vi "SUB_Parsing_from_table_to_cluster.vi"(0 "ROM Table":string[][](table)=[["Device ID", "4294967295", "MAX Value: 4294967295 (FFFFFFFFh)"], ["YEAR", "255", "Year: 2255, MAX Value: 255 (FFh)"], ["Month", "255", "Month: 255, MAX Value: 255 (FFh)"], ["Day", "255", "Day: 255, MAX Value: 255 (FFh)"], ["Device Type", "65535", "-"], ["Manufacturer ID", "4294967295", "MAX Value: 4294967295 (FFFFFFFFh)"], ["Cal_Scale A", "0", "MAX Value: 255 (FF)"], ["Cal_Scale B", "0", "MAX Value: 255 (FF)"], ["Cal_Acc. X", "0", "-"], ["Cal_Acc. Y", "0", "-"], ["Cal_Acc. Z", "0", "-"], ["Cal_Gy. X", "0", "-"], ["Cal_Gy. Y", "0", "-"], ["Cal_Gy. Z", "0", "-"], ["Cal_Vol H", "0", "-"], ["Cal_Vol L", "0", "-"], ["Cal_CDC Off 1", "0", "-"], ["Cal_CDC Off 2", "0", "-"], ["Cal_CDC Off 3", "0", "-"], ["Cal_CDC Off 4", "0", "-"], ["Cal_CDC Off 5", "0", "-"], ["Cal_CDC Off 6", "0", "-"], ["Cal_CDC Off 7", "0", "-"], ["Cal_CDC Off 8", "0", "-"], ["Firmware Revision", "-", "-"], ["Operative Side", "-", "-"], ["Cal_Compart. A_10", "-", "-"], ["Cal_Compart. B_10", "-", "-"], ["Reserved", "-", "-"], ["Cal_Compart. A_11", "-", "-"], ["Cal_Compart. B_11", "-", "-"], ["Cal_Compart. A_12", "-", "-"], ["Cal_Compart. B_12", "-", "-"], ["Cal_Compart. A_13", "-", "-"], ["Cal_Compart. B_13", "-", "-"], ["Cal_Compart. A_14", "-", "-"], ["Cal_Compart. B_14", "-", "-"], ["Cal_Compart. A_16", "-", "-"], ["Cal_Compart. B_16", "-", "-"], ["Reserved", "-", "-"], ["Acc. X_0 value", "-", "-"], ["Acc. Y_0 value", "-", "-"], ["Acc. Z_0 value", "-", "-"], ["Acc. X_45 value", "-", "-"], ["Acc. Y_45 value", "-", "-"], ["Acc. Z_45 value", "-", "-"], ["Reserved", "-", "-"], ["Acc. X_90 value", "-", "-"], ["Acc. Y_90 value", "-", "-"], ["Acc. Z_90 value", "-", "-"], ["Acc. X_180 value", "-", "-"], ["Acc. Y_180 value", "-", "-"], ["Acc. Z_180 value", "-", "-"], ["Reserved", "-", "-"], ["", "", ""], ["", "", ""], ["", "", ""], ["", "", ""], ["", "", ""], ["", "", ""], ["", "", ""], ["", "", ""], ["", "", ""], ["", "", ""], ["", "", ""], ["", "", ""], ["", "", ""], ["", "", ""], ["", "", ""]]) -> (11 "Acclerometer value(90, 180)":T1 {"Check sum" format="%x"; "Reserved_2" format="%x"; "Reserved_1" format="%x"; "second counter_2" format="%x"; "Acc. Z_90 val_L" format="%x"; "second counter_1" format="%x"; "Acc. Z_180 val_L" format="%x"; "Acc. Z_180 val_H" format="%x"; "Acc. Y_180 val_L" format="%x"; "Acc. Y_180 val_H" format="%x"; "Acc. X_180 val_L" format="%x"; "Acc. X_180 val_H" format="%x"; "Acc. Z_90 val_H" format="%x"; "Acc. Y_90 val_L" format="%x"; "Acc. Y_90 val_H" format="%x"; "Acc. X_90 val_L" format="%x"; "Acc. X_90 val_H" format="%x"; "Packet ID" format="%x"}, 12 "data4":T3 {"Check sum" format="%x"; "Reserved_8" format="%x"; "Reserved_7" format="%x"; "Reserved_6" format="%x"; "Cal_Compart. B_16_2" format="%x"; "Reserved_5" format="%x"; "Reserved_4" format="%x"; "Reserved_3" format="%x"; "Reserved_2" format="%x"; "Reserved_1" format="%x"; "Cal_Compart. B_16_4" format="%x"; "Cal_Compart. B_16_3" format="%x"; "Cal_Compart. B_16_1" format="%x"; "Cal_Compart. A_16_4" format="%x"; "Cal_Compart. A_16_3" format="%x"; "Cal_Compart. A_16_2" format="%x"; "Cal_Compart. A_16_1" format="%x"; "Packet ID" format="%x"}, 13 "Acclerometer value(0, 45)":T2 {"Check sum" format="%x"; "Reserved_4" format="%x"; "Reserved_3" format="%x"; "Reserved_2" format="%x"; "Acc. Z_0 val_L" format="%x"; "Reserved_1" format="%x"; "Acc. Z_45 val_L" format="%x"; "Acc. Z_45 val_H" format="%x"; "Acc. Y_45 val_L" format="%x"; "Acc. Y_45 val_H" format="%x"; "Acc. X_45 val_L" format="%x"; "Acc. X_45 val_H" format="%x"; "Acc. Z_0 val_H" format="%x"; "Acc. Y_0 val_L" format="%x"; "Acc. Y_0 val_H" format="%x"; "Acc. X_0 val_L" format="%x"; "Acc. X_0 val_H" format="%x"; "Packet ID" format="%x"}, 14 "Device information":T7 {"Check sum 2" format="%x"; "Device Type L" format="%x"; "Device Type H" format="%x"; "Check sum" format="%x"; "Scale B" format="%x"; "Scale A" format="%x"; "Manufacturer Lot ID 4" format="%x"; "Manufacturer Lot ID 3" format="%x"; "Manufacturer Lot ID 2" format="%x"; "Manufacturer Lot ID 1" format="%x"; "Day" format="%x"; "Month" format="%x"; "Year" format="%x"; "Device ID 4" format="%x"; "Device ID 3" format="%x"; "Device ID 2" format="%x"; "Device ID 1" format="%x"; "Packet ID" format="%x"}, 15 "Cal information":T9 {"Check sum" format="%x"; "Voltage L 2.8V" format="%x"; "Voltage H 2.8V" format="%x"; "Voltage L 3.1V" format="%x"; "Acc Z_L_Cal" format="%x"; "Voltage H 3.1V" format="%x"; "Gyro Z_L_Cal" format="%x"; "Gyro Z_H_Cal" format="%x"; "Gyro Y_L_Cal" format="%x"; "Gyro Y_H_Cal" format="%x"; "Gyro X_L_Cal" format="%x"; "Gyro X_H_Cal" format="%x"; "Acc Z_H_Cal" format="%x"; "Acc Y_L_Cal" format="%x"; "Acc Y_H_Cal" format="%x"; "Acc X_L_Cal" format="%x"; "Acc X_H_Cal" format="%x"; "Packet ID" format="%x"}, 16 "PCAP zero information":T8 {"Check sum" format="%x"; "Sensor 8_L" format="%x"; "Sensor 8_H" format="%x"; "Sensor 7_L" format="%x"; "Sensor 7_H" format="%x"; "Sensor 6_L" format="%x"; "Sensor 6_H" format="%x"; "Sensor 5_L" format="%x"; "Sensor 5_H" format="%x"; "Sensor 4_L" format="%x"; "Sensor 4_H" format="%x"; "Sensor 3_L" format="%x"; "Sensor 3_H" format="%x"; "Sensor 2_L" format="%x"; "Sensor 2_H" format="%x"; "Sensor 1_L" format="%x"; "Sensor 1_H" format="%x"; "Packet ID" format="%x"}, 17 "data1":T6 {"Check sum" format="%x"; "Reserved_6" format="%x"; "Reserved_5" format="%x"; "Reserved_4" format="%x"; "Cal_Compart. A_10_4" format="%x"; "Reserved_3" format="%x"; "Reserved_2" format="%x"; "Reserved_1" format="%x"; "Cal_Compart. B_10_4" format="%x"; "Cal_Compart. B_10_3" format="%x"; "Cal_Compart. B_10_2" format="%x"; "Cal_Compart. B_10_1" format="%x"; "Cal_Compart. A_10_3" format="%x"; "Cal_Compart. A_10_2" format="%x"; "Cal_Compart. A_10_1" format="%x"; "Operative Side" format="%x"; "Firmware Revision" format="%x"; "Packet ID" format="%x"}, 18 "data2":T5 {"Check sum" format="%x"; "Cal_Compart. B_12_4" format="%x"; "Cal_Compart. B_12_3" format="%x"; "Cal_Compart. B_12_2" format="%x"; "Cal_Compart. B_11_2" format="%x"; "Cal_Compart. B_12_1" format="%x"; "Cal_Compart. A_12_4" format="%x"; "Cal_Compart. A_12_3" format="%x"; "Cal_Compart. A_12_2" format="%x"; "Cal_Compart. A_12_1" format="%x"; "Cal_Compart. B_11_4" format="%x"; "Cal_Compart. B_11_3" format="%x"; "Cal_Compart. B_11_1" format="%x"; "Cal_Compart. A_11_4" format="%x"; "Cal_Compart. A_11_3" format="%x"; "Cal_Compart. A_11_2" format="%x"; "Cal_Compart. A_11_1" format="%x"; "Packet ID" format="%x"}, 19 "data3":T4 {"Check sum" format="%x"; "Cal_Compart. B_14_4" format="%x"; "Cal_Compart. B_14_3" format="%x"; "Cal_Compart. B_14_2" format="%x"; "Cal_Compart. B_13_2" format="%x"; "Cal_Compart. B_14_1" format="%x"; "Cal_Compart. A_14_4" format="%x"; "Cal_Compart. A_14_3" format="%x"; "Cal_Compart. A_14_2" format="%x"; "Cal_Compart. A_14_1" format="%x"; "Cal_Compart. B_13_4" format="%x"; "Cal_Compart. B_13_3" format="%x"; "Cal_Compart. B_13_1" format="%x"; "Cal_Compart. A_13_4" format="%x"; "Cal_Compart. A_13_3" format="%x"; "Cal_Compart. A_13_2" format="%x"; "Cal_Compart. A_13_1" format="%x"; "Packet ID" format="%x"})   [LabVIEW 2015]
uses:
  Cluster Type/Cal information.ctl
  Cluster Type/PCAP zero information.ctl
  Cluster Type/Device information.ctl
  Cluster Type/add data1.ctl
  Cluster Type/add data2.ctl
  Cluster Type/add data3.ctl
  Cluster Type/add data4.ctl
  Cluster Type/Acclerometer value(0, 45).ctl
  Cluster Type/Acclerometer value(90, 180).ctl
panel:
  out "32비트 정수":u8
  out "32비트 정수 2":u8
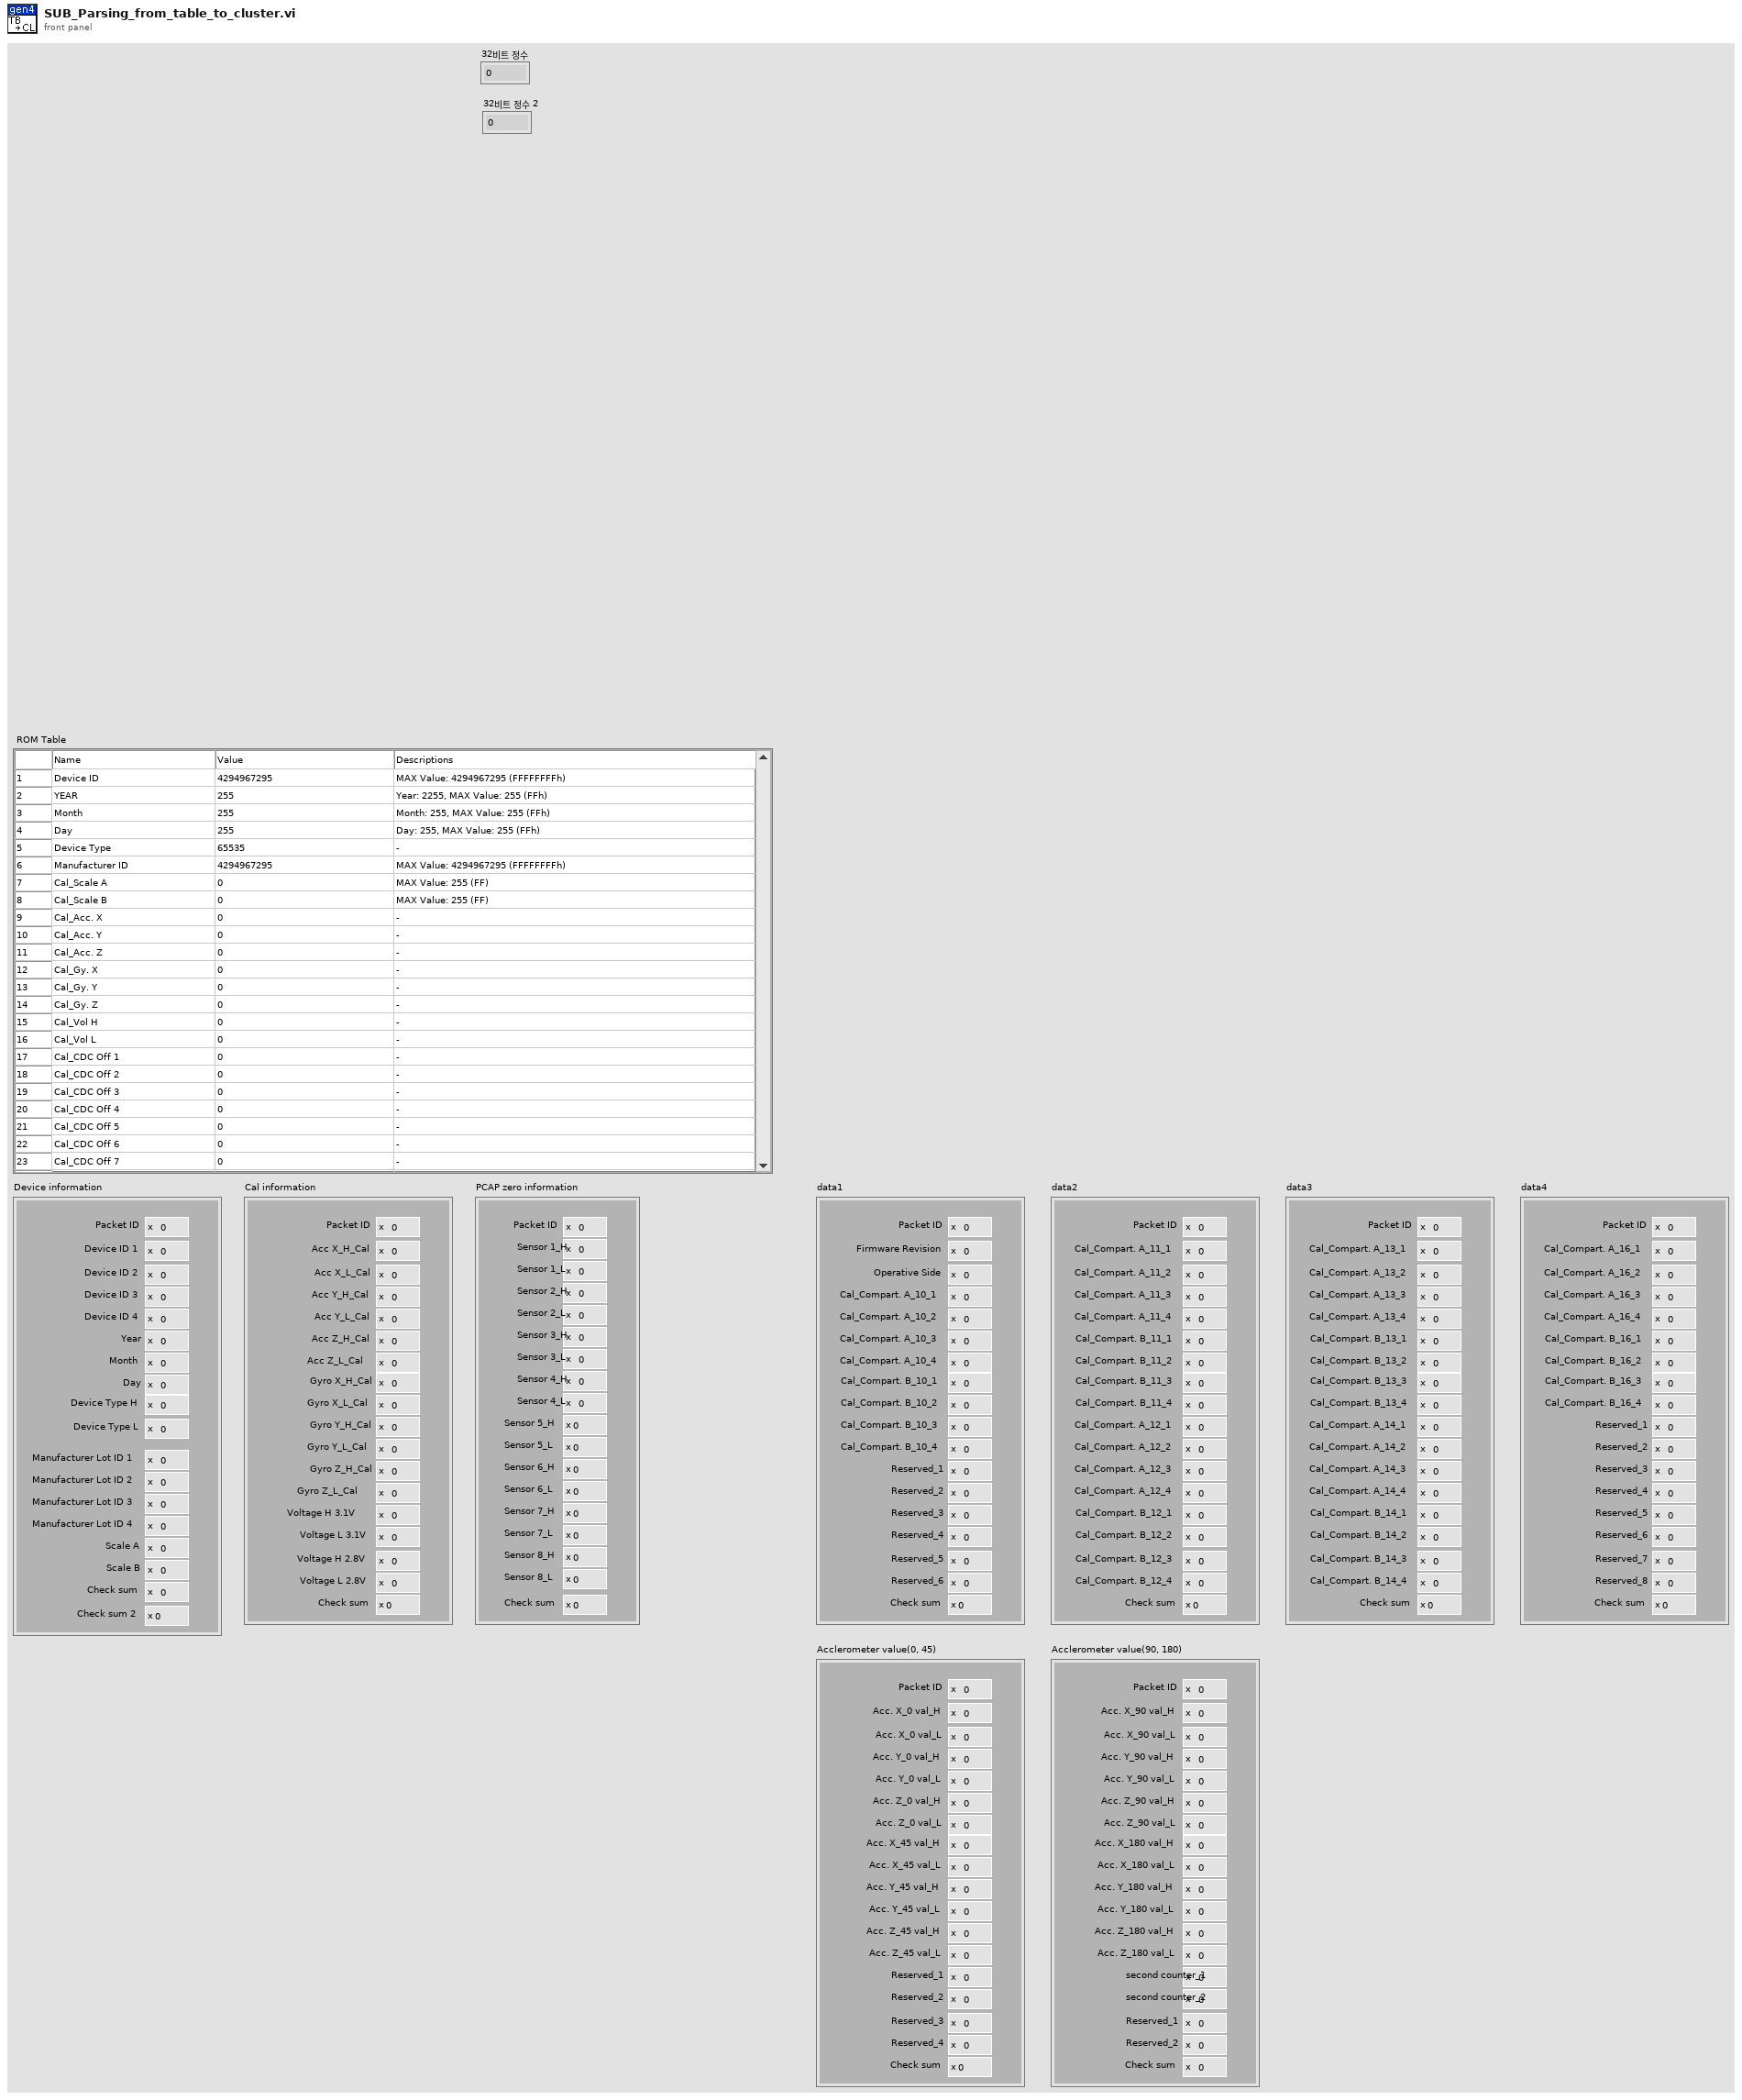
[diagram p1: front panel]
types:
  T1 = typedef "Acclerometer value(90, 180).ctl" = cluster{"Packet ID":u8, "Acc. X_90 val_H":u8, "Acc. X_90 val_L":u8, "Acc. Y_90 val_H":u8, "Acc. Y_90 val_L":u8, "Acc. Z_90 val_H":u8, "Acc. Z_90 val_L":u8, "Acc. X_180 val_H":u8, "Acc. X_180 val_L":u8, "Acc. Y_180 val_H":u8, "Acc. Y_180 val_L":u8, "Acc. Z_180 val_H":u8, "Acc. Z_180 val_L":u8, "second counter_1":u8, "second counter_2":u8, "Reserved_1":u8, "Reserved_2":u8, "Check sum":u8}
  T2 = typedef "Acclerometer value(0, 45).ctl" = cluster{"Packet ID":u8, "Acc. X_0 val_H":u8, "Acc. X_0 val_L":u8, "Acc. Y_0 val_H":u8, "Acc. Y_0 val_L":u8, "Acc. Z_0 val_H":u8, "Acc. Z_0 val_L":u8, "Acc. X_45 val_H":u8, "Acc. X_45 val_L":u8, "Acc. Y_45 val_H":u8, "Acc. Y_45 val_L":u8, "Acc. Z_45 val_H":u8, "Acc. Z_45 val_L":u8, "Reserved_1":u8, "Reserved_2":u8, "Reserved_3":u8, "Reserved_4":u8, "Check sum":u8}
  T3 = typedef "add data4.ctl" = cluster{"Packet ID":u8, "Cal_Compart. A_16_1":u8, "Cal_Compart. A_16_2":u8, "Cal_Compart. A_16_3":u8, "Cal_Compart. A_16_4":u8, "Cal_Compart. B_16_1":u8, "Cal_Compart. B_16_2":u8, "Cal_Compart. B_16_3":u8, "Cal_Compart. B_16_4":u8, "Reserved_1":u8, "Reserved_2":u8, "Reserved_3":u8, "Reserved_4":u8, "Reserved_5":u8, "Reserved_6":u8, "Reserved_7":u8, "Reserved_8":u8, "Check sum":u8}
  T4 = typedef "add data3.ctl" = cluster{"Packet ID":u8, "Cal_Compart. A_13_1":u8, "Cal_Compart. A_13_2":u8, "Cal_Compart. A_13_3":u8, "Cal_Compart. A_13_4":u8, "Cal_Compart. B_13_1":u8, "Cal_Compart. B_13_2":u8, "Cal_Compart. B_13_3":u8, "Cal_Compart. B_13_4":u8, "Cal_Compart. A_14_1":u8, "Cal_Compart. A_14_2":u8, "Cal_Compart. A_14_3":u8, "Cal_Compart. A_14_4":u8, "Cal_Compart. B_14_1":u8, "Cal_Compart. B_14_2":u8, "Cal_Compart. B_14_3":u8, "Cal_Compart. B_14_4":u8, "Check sum":u8}
  T5 = typedef "add data2.ctl" = cluster{"Packet ID":u8, "Cal_Compart. A_11_1":u8, "Cal_Compart. A_11_2":u8, "Cal_Compart. A_11_3":u8, "Cal_Compart. A_11_4":u8, "Cal_Compart. B_11_1":u8, "Cal_Compart. B_11_2":u8, "Cal_Compart. B_11_3":u8, "Cal_Compart. B_11_4":u8, "Cal_Compart. A_12_1":u8, "Cal_Compart. A_12_2":u8, "Cal_Compart. A_12_3":u8, "Cal_Compart. A_12_4":u8, "Cal_Compart. B_12_1":u8, "Cal_Compart. B_12_2":u8, "Cal_Compart. B_12_3":u8, "Cal_Compart. B_12_4":u8, "Check sum":u8}
  T6 = typedef "add data1.ctl" = cluster{"Packet ID":u8, "Firmware Revision":u8, "Operative Side":u8, "Cal_Compart. A_10_1":u8, "Cal_Compart. A_10_2":u8, "Cal_Compart. A_10_3":u8, "Cal_Compart. A_10_4":u8, "Cal_Compart. B_10_1":u8, "Cal_Compart. B_10_2":u8, "Cal_Compart. B_10_3":u8, "Cal_Compart. B_10_4":u8, "Reserved_1":u8, "Reserved_2":u8, "Reserved_3":u8, "Reserved_4":u8, "Reserved_5":u8, "Reserved_6":u8, "Check sum":u8}
  T7 = typedef "Device information.ctl" = cluster{"Packet ID":u8, "Device ID 1":u8, "Device ID 2":u8, "Device ID 3":u8, "Device ID 4":u8, "Year":u8, "Month":u8, "Day":u8, "Device Type H":u8, "Device Type L":u8, "Manufacturer Lot ID 1":u8, "Manufacturer Lot ID 2":u8, "Manufacturer Lot ID 3":u8, "Manufacturer Lot ID 4":u8, "Scale A":u8, "Scale B":u8, "Check sum":u8, "Check sum 2":u8}
  T8 = typedef "PCAP zero information.ctl" = cluster{"Packet ID":u8, "Sensor 1_H":u8, "Sensor 1_L":u8, "Sensor 2_H":u8, "Sensor 2_L ":u8, "Sensor 3_H":u8, "Sensor 3_L":u8, "Sensor 4_H":u8, "Sensor 4_L":u8, "Sensor 5_H":u8, "Sensor 5_L":u8, "Sensor 6_H":u8, "Sensor 6_L":u8, "Sensor 7_H":u8, "Sensor 7_L":u8, "Sensor 8_H":u8, "Sensor 8_L":u8, "Check sum":u8}
  T9 = typedef "Cal information.ctl" = cluster{"Packet ID":u8, "Acc X_H_Cal":u8, "Acc X_L_Cal":u8, "Acc Y_H_Cal":u8, "Acc Y_L_Cal":u8, "Acc Z_H_Cal":u8, "Acc Z_L_Cal":u8, "Gyro X_H_Cal":u8, "Gyro X_L_Cal":u8, "Gyro Y_H_Cal":u8, "Gyro Y_L_Cal":u8, "Gyro Z_H_Cal":u8, "Gyro Z_L_Cal":u8, "Voltage H 3.1V":u8, "Voltage L 3.1V":u8, "Voltage H 2.8V":u8, "Voltage L 2.8V":u8, "Check sum":u8}
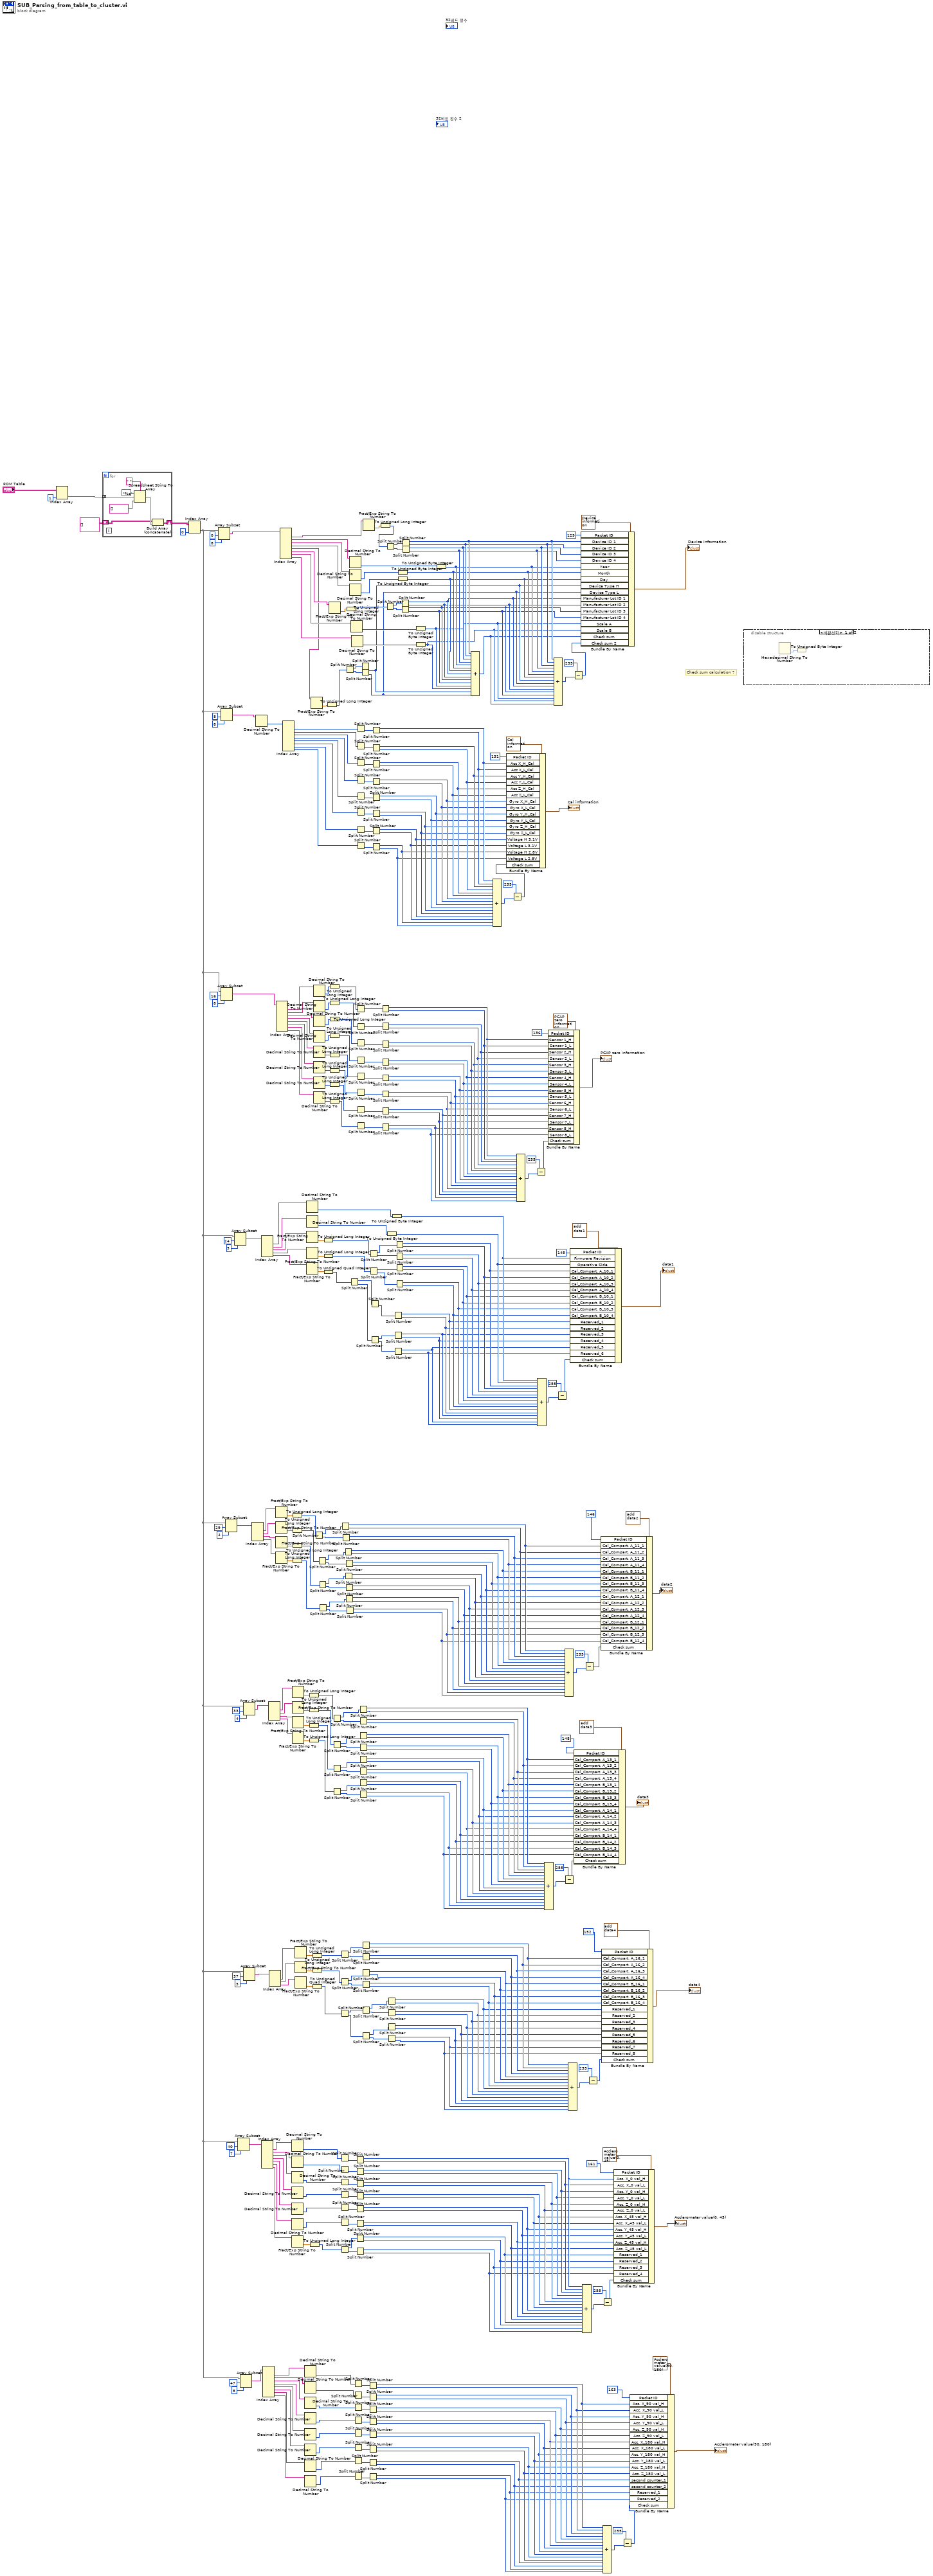
[diagram p0: block diagram]
diagram:
  # "Check sum calculation ?"
  n1 = Index Array(array="ROM Table", index (col)=1 ("비활성화된 인덱스 (열)")) -> (element=w388:string[])  [unwired: 1 in]
  n2 = for {
    tunnel: w388 -> [w441] mode=indexing
    shift-right: [w436] -> w385
    shift-left: string[][] [] -> [w435]
    n3 = Spreadsheet String To Array(delimiter (Tab)=" " ("구분 문자(탭)"), format string="%s" ("포맷 문자열"), spreadsheet string=w441, array type (2D Dbl)=string[] []) -> (array=w437:string[])
    n4 = Build Array (concatenate)(w435, w437) -> (w436:string[][])
  }
  n5 = Index Array(array=w385, index (col)=0 ("비활성화된 인덱스 (열)")) -> (element=w313:string[])  [unwired: 1 in]
  n6 = Array Subset(array=w313, index=0 ("인덱스"), length=8 ("길이")) -> (w417:string[])
  n7 = Array Subset(array=w313, index=8 ("인덱스"), length=8 ("길이")) -> (w412:string[])
  n8 = Array Subset(array=w313, index=16 ("인덱스"), length=8 ("길이")) -> (w236:string[])
  n9 = Array Subset(array=w313, index=29 ("인덱스"), length=4 ("길이")) -> (w196:string[])
  n10 = Array Subset(array=w313, index=24 ("인덱스"), length=5 ("길이")) -> (w227:string[])
  n11 = Array Subset(array=w313, index=40 ("인덱스"), length=7 ("길이")) -> (w81:string[])
  n12 = Array Subset(array=w313, index=47 ("인덱스"), length=8 ("길이")) -> (w28:string[])
  n13 = Array Subset(array=w313, index=33 ("인덱스"), length=4 ("길이")) -> (w156:string[])
  n14 = Array Subset(array=w313, index=37 ("인덱스"), length=3 ("길이")) -> (w130:string[])
  n15 = Index Array(array=w196) -> (element #1=w191:string, element #2=w190:string, element #3=w189:string, element #4=w188:string)  [unwired: 4 in]
  n16 = Decimal String To Number(string=w412) -> (number=w411:i32[])  [unwired: 2 in, 1 out]
  n17 = Index Array(array=w227) -> (element #1=w226:string, element #2=w225:string, element #3=w85:string, element #4=w84:string, element #5=w222:string)  [unwired: 5 in]
  n18 = Index Array(array=w81) -> (element #1=w80:string, element #2=w79:string, element #3=w78:string, element #4=w77:string, element #5=w76:string, element #6=w75:string, element #7=w73:string)  [unwired: 7 in]
  n19 = Index Array(array=w28) -> (element #1=w40:string, element #2=w39:string, element #3=w38:string, element #4=w37:string, element #5=w36:string, element #6=w35:string, element #7=w12:string, element #8=w11:string)  [unwired: 8 in]
  n20 = Index Array(array=w156) -> (element #1=w160:string, element #2=w159:string, element #3=w158:string, element #4=w157:string)  [unwired: 4 in]
  n21 = Index Array(array=w130) -> (element #1=w129:string, element #2=w128:string, element #3=w126:string)  [unwired: 3 in]
  n22 = Fract/Exp String To Number(string=w191) -> (number=w194:dbl)  [unwired: 3 in, 1 out]
  n23 = Fract/Exp String To Number(string=w190) -> (number=w195:dbl)  [unwired: 3 in, 1 out]
  n24 = Fract/Exp String To Number(string=w189) -> (number=w193:dbl)  [unwired: 3 in, 1 out]
  n25 = Fract/Exp String To Number(string=w188) -> (number=w192:dbl)  [unwired: 3 in, 1 out]
  n26 = Index Array(array=w236) -> (element #1=w235:string, element #2=w234:string, element #3=w233:string, element #4=w232:string, element #5=w231:string, element #6=w230:string, element #7=w229:string, element #8=w228:string)  [unwired: 8 in]
  n27 = Index Array(array=w417) -> (element #1=w378:string, element #2=w426:string, element #3=w425:string, element #4=w424:string, element #5=w372:string, element #6=w375:string, element #7=w383:string, element #8=w382:string)  [unwired: 8 in]
  n28 = Index Array(array=w411) -> (element #1=w410:i32, element #2=w404:i32, element #3=w403:i32, element #4=w400:i32, element #5=w399:i32, element #6=w398:i32, element #7=w397:i32, element #8=w396:i32)  [unwired: 8 in]
  n29 = To Unsigned Long Integer(number=w194) -> (unsigned 32bit integer=w187:u32)
  n30 = To Unsigned Long Integer(number=w195) -> (unsigned 32bit integer=w186:u32)
  n31 = To Unsigned Long Integer(number=w193) -> (unsigned 32bit integer=w185:u32)
  n32 = To Unsigned Long Integer(number=w192) -> (unsigned 32bit integer=w184:u32)
  n33 = Decimal String To Number(string=w80) -> (number=w72:i32)  [unwired: 2 in, 1 out]
  n34 = Decimal String To Number(string=w79) -> (number=w71:i32)  [unwired: 2 in, 1 out]
  n35 = Decimal String To Number(string=w78) -> (number=w70:i32)  [unwired: 2 in, 1 out]
  n36 = Decimal String To Number(string=w77) -> (number=w69:i32)  [unwired: 2 in, 1 out]
  n37 = Decimal String To Number(string=w76) -> (number=w68:i32)  [unwired: 2 in, 1 out]
  n38 = Decimal String To Number(string=w75) -> (number=w67:i32)  [unwired: 2 in, 1 out]
  n39 = Fract/Exp String To Number(string=w73) -> (number=w74:dbl)  [unwired: 3 in, 1 out]
  n40 = Fract/Exp String To Number(string=w160) -> (number=w163:dbl)  [unwired: 3 in, 1 out]
  n41 = Fract/Exp String To Number(string=w159) -> (number=w164:dbl)  [unwired: 3 in, 1 out]
  n42 = Fract/Exp String To Number(string=w158) -> (number=w162:dbl)  [unwired: 3 in, 1 out]
  n43 = Fract/Exp String To Number(string=w157) -> (number=w161:dbl)  [unwired: 3 in, 1 out]
  n44 = Fract/Exp String To Number(string=w129) -> (number=w131:dbl)  [unwired: 3 in, 1 out]
  n45 = Fract/Exp String To Number(string=w128) -> (number=w132:dbl)  [unwired: 3 in, 1 out]
  n46 = Fract/Exp String To Number(string=w126) -> (number=w127:dbl)  [unwired: 3 in, 1 out]
  n47 = Decimal String To Number(string=w40) -> (number=w34:i32)  [unwired: 2 in, 1 out]
  n48 = Decimal String To Number(string=w39) -> (number=w33:i32)  [unwired: 2 in, 1 out]
  n49 = Decimal String To Number(string=w38) -> (number=w32:i32)  [unwired: 2 in, 1 out]
  n50 = Decimal String To Number(string=w37) -> (number=w31:i32)  [unwired: 2 in, 1 out]
  n51 = Decimal String To Number(string=w36) -> (number=w30:i32)  [unwired: 2 in, 1 out]
  n52 = Decimal String To Number(string=w35) -> (number=w29:i32)  [unwired: 2 in, 1 out]
  n53 = Decimal String To Number(string=w12) -> (number=w10:i32)  [unwired: 2 in, 1 out]
  n54 = Decimal String To Number(string=w11) -> (number=w9:i32)  [unwired: 2 in, 1 out]
  n55 = Decimal String To Number(string=w226) -> (number=w224:i32)  [unwired: 2 in, 1 out]
  n56 = Decimal String To Number(string=w225) -> (number=w223:i32)  [unwired: 2 in, 1 out]
  n57 = Fract/Exp String To Number(string=w85) -> (number=w87:dbl)  [unwired: 3 in, 1 out]
  n58 = Fract/Exp String To Number(string=w84) -> (number=w86:dbl)  [unwired: 3 in, 1 out]
  n59 = Fract/Exp String To Number(string=w222) -> (number=w221:dbl)  [unwired: 3 in, 1 out]
  n60 = To Unsigned Long Integer(number=w163) -> (unsigned 32bit integer=w155:u32)
  n61 = To Unsigned Long Integer(number=w164) -> (unsigned 32bit integer=w154:u32)
  n62 = To Unsigned Long Integer(number=w162) -> (unsigned 32bit integer=w153:u32)
  n63 = To Unsigned Long Integer(number=w161) -> (unsigned 32bit integer=w152:u32)
  n64 = To Unsigned Long Integer(number=w74) -> (unsigned 32bit integer=w66:u32)
  n65 = Fract/Exp String To Number(string=w372) -> (number=w373:dbl)  [unwired: 3 in, 1 out]
  n66 = To Unsigned Long Integer(number=w131) -> (unsigned 32bit integer=w125:u32)
  n67 = To Unsigned Long Integer(number=w132) -> (unsigned 32bit integer=w124:u32)
  n68 = To Unsigned Quad Integer(1:w127) -> (0:w123:u64)
  n69 = Decimal String To Number(string=w235) -> (number=w103:i32)  [unwired: 2 in, 1 out]
  n70 = Decimal String To Number(string=w234) -> (number=w102:i32)  [unwired: 2 in, 1 out]
  n71 = Decimal String To Number(string=w233) -> (number=w101:i32)  [unwired: 2 in, 1 out]
  n72 = Decimal String To Number(string=w232) -> (number=w100:i32)  [unwired: 2 in, 1 out]
  n73 = Decimal String To Number(string=w231) -> (number=w99:i32)  [unwired: 2 in, 1 out]
  n74 = Decimal String To Number(string=w230) -> (number=w98:i32)  [unwired: 2 in, 1 out]
  n75 = Decimal String To Number(string=w229) -> (number=w97:i32)  [unwired: 2 in, 1 out]
  n76 = Decimal String To Number(string=w228) -> (number=w96:i32)  [unwired: 2 in, 1 out]
  n77 = Split Number(x=w187) -> (hi(x)=w358:u16, lo(x)=w359:u16)
  n78 = Split Number(x=w186) -> (hi(x)=w355:u16, lo(x)=w356:u16)
  n79 = Split Number(x=w185) -> (hi(x)=w353:u16, lo(x)=w354:u16)
  n80 = Split Number(x=w184) -> (hi(x)=w351:u16, lo(x)=w352:u16)
  n81 = To Unsigned Long Integer(number=w87) -> (unsigned 32bit integer=w83:u32)
  n82 = To Unsigned Long Integer(number=w86) -> (unsigned 32bit integer=w82:u32)
  n83 = To Unsigned Quad Integer(1:w221) -> (0:w220:u64)
  n84 = To Unsigned Long Integer(number=w373) -> (unsigned 32bit integer=w371:u32)
  n85 = Fract/Exp String To Number(string=w375) -> (number=w376:dbl)  [unwired: 3 in, 1 out]
  n86 = To Unsigned Long Integer(number=w103) -> (unsigned 32bit integer=w95:u32)
  n87 = To Unsigned Long Integer(number=w102) -> (unsigned 32bit integer=w94:u32)
  n88 = To Unsigned Long Integer(number=w101) -> (unsigned 32bit integer=w93:u32)
  n89 = To Unsigned Long Integer(number=w100) -> (unsigned 32bit integer=w92:u32)
  n90 = To Unsigned Long Integer(number=w99) -> (unsigned 32bit integer=w91:u32)
  n91 = To Unsigned Long Integer(number=w98) -> (unsigned 32bit integer=w90:u32)
  n92 = To Unsigned Long Integer(number=w97) -> (unsigned 32bit integer=w89:u32)
  n93 = To Unsigned Long Integer(number=w96) -> (unsigned 32bit integer=w88:u32)
  n94 = Split Number(x=w155) -> (hi(x)=w346:u16, lo(x)=w347:u16)
  n95 = Split Number(x=w154) -> (hi(x)=w344:u16, lo(x)=w345:u16)
  n96 = Split Number(x=w153) -> (hi(x)=w342:u16, lo(x)=w343:u16)
  n97 = Split Number(x=w152) -> (hi(x)=w340:u16, lo(x)=w341:u16)
  n98 = Split Number(x=w125) -> (hi(x)=w335:u16, lo(x)=w336:u16)
  n99 = Split Number(x=w124) -> (hi(x)=w333:u16, lo(x)=w334:u16)
  n100 = Split Number(x=w123) -> (hi(x)=w330:u32, lo(x)=w327:u32)
  n101 = Split Number(x=w72) -> (lo(x)=w323:u16)  [unwired: 1 out]
  n102 = Split Number(x=w71) -> (lo(x)=w322:u16)  [unwired: 1 out]
  n103 = Split Number(x=w70) -> (lo(x)=w321:u16)  [unwired: 1 out]
  n104 = Split Number(x=w69) -> (lo(x)=w320:u16)  [unwired: 1 out]
  n105 = Split Number(x=w68) -> (lo(x)=w319:u16)  [unwired: 1 out]
  n106 = Split Number(x=w67) -> (lo(x)=w318:u16)  [unwired: 1 out]
  n107 = Split Number(x=w66) -> (hi(x)=w316:u16, lo(x)=w317:u16)
  n108 = Split Number(x=w358) -> (hi(x)=w180:u8, lo(x)=w179:u8)
  n109 = Split Number(x=w359) -> (hi(x)=w178:u8, lo(x)=w177:u8)
  n110 = Split Number(x=w355) -> (hi(x)=w176:u8, lo(x)=w175:u8)
  n111 = Split Number(x=w353) -> (hi(x)=w172:u8, lo(x)=w171:u8)
  n112 = Split Number(x=w356) -> (hi(x)=w174:u8, lo(x)=w173:u8)
  n113 = Split Number(x=w351) -> (hi(x)=w168:u8, lo(x)=w167:u8)
  n114 = Split Number(x=w354) -> (hi(x)=w170:u8, lo(x)=w169:u8)
  n115 = Split Number(x=w371) -> (hi(x)=w421:u16, lo(x)=w420:u16)
  n116 = Split Number(x=w352) -> (hi(x)=w166:u8, lo(x)=w165:u8)
  n117 = To Unsigned Long Integer(number=w376) -> (unsigned 32bit integer=w374:u32)
  n118 = Split Number(x=w220) -> (hi(x)=w217:u32, lo(x)=w216:u32)
  n119 = Decimal String To Number(string=w426) -> (number=w384:i32)  [unwired: 2 in, 1 out]
  n120 = Decimal String To Number(string=w425) -> (number=w423:i32)  [unwired: 2 in, 1 out]
  n121 = Decimal String To Number(string=w424) -> (number=w422:i32)  [unwired: 2 in, 1 out]
  n122 = Decimal String To Number(string=w383) -> (number=w381:i32)  [unwired: 2 in, 1 out]
  n123 = Decimal String To Number(string=w382) -> (number=w380:i32)  [unwired: 2 in, 1 out]
  n124 = Split Number(x=w34) -> (lo(x)=w46:u16)  [unwired: 1 out]
  n125 = Split Number(x=w33) -> (lo(x)=w45:u16)  [unwired: 1 out]
  n126 = Split Number(x=w32) -> (lo(x)=w44:u16)  [unwired: 1 out]
  n127 = Split Number(x=w31) -> (lo(x)=w43:u16)  [unwired: 1 out]
  n128 = Split Number(x=w30) -> (lo(x)=w42:u16)  [unwired: 1 out]
  n129 = Split Number(x=w29) -> (lo(x)=w41:u16)  [unwired: 1 out]
  n130 = Split Number(x=w10) -> (lo(x)=w8:u16)  [unwired: 1 out]
  n131 = Split Number(x=w9) -> (lo(x)=w7:u16)  [unwired: 1 out]
  n132 = Split Number(x=w323) -> (hi(x)=w62:u8, lo(x)=w61:u8)
  n133 = Split Number(x=w322) -> (hi(x)=w60:u8, lo(x)=w59:u8)
  n134 = Split Number(x=w321) -> (hi(x)=w58:u8, lo(x)=w57:u8)
  n135 = Split Number(x=w320) -> (hi(x)=w56:u8, lo(x)=w55:u8)
  n136 = Split Number(x=w319) -> (hi(x)=w54:u8, lo(x)=w53:u8)
  n137 = Split Number(x=w318) -> (hi(x)=w52:u8, lo(x)=w51:u8)
  n138 = Split Number(x=w316) -> (hi(x)=w50:u8, lo(x)=w49:u8)
  n139 = Split Number(x=w317) -> (hi(x)=w48:u8, lo(x)=w47:u8)
  n140 = Split Number(x=w410) -> (lo(x)=w413:u16)  [unwired: 1 out]
  n141 = Split Number(x=w404) -> (lo(x)=w409:u16)  [unwired: 1 out]
  n142 = Split Number(x=w403) -> (lo(x)=w408:u16)  [unwired: 1 out]
  n143 = Split Number(x=w400) -> (lo(x)=w407:u16)  [unwired: 1 out]
  n144 = Split Number(x=w399) -> (lo(x)=w406:u16)  [unwired: 1 out]
  n145 = Split Number(x=w398) -> (lo(x)=w405:u16)  [unwired: 1 out]
  n146 = Split Number(x=w397) -> (lo(x)=w401:u16)  [unwired: 1 out]
  n147 = Split Number(x=w396) -> (lo(x)=w402:u16)  [unwired: 1 out]
  n148 = Split Number(x=w95) -> (lo(x)=w264:u16)  [unwired: 1 out]
  n149 = Split Number(x=w94) -> (lo(x)=w263:u16)  [unwired: 1 out]
  n150 = Split Number(x=w93) -> (lo(x)=w262:u16)  [unwired: 1 out]
  n151 = Split Number(x=w92) -> (lo(x)=w261:u16)  [unwired: 1 out]
  n152 = Split Number(x=w91) -> (lo(x)=w260:u16)  [unwired: 1 out]
  n153 = Split Number(x=w90) -> (lo(x)=w259:u16)  [unwired: 1 out]
  n154 = Split Number(x=w89) -> (lo(x)=w258:u16)  [unwired: 1 out]
  n155 = Split Number(x=w88) -> (lo(x)=w257:u16)  [unwired: 1 out]
  n156 = Split Number(x=w346) -> (hi(x)=w148:u8, lo(x)=w147:u8)
  n157 = Split Number(x=w347) -> (hi(x)=w146:u8, lo(x)=w145:u8)
  n158 = Split Number(x=w344) -> (hi(x)=w144:u8, lo(x)=w143:u8)
  n159 = Split Number(x=w345) -> (hi(x)=w142:u8, lo(x)=w141:u8)
  n160 = Split Number(x=w342) -> (hi(x)=w140:u8, lo(x)=w139:u8)
  n161 = Split Number(x=w343) -> (hi(x)=w138:u8, lo(x)=w137:u8)
  n162 = Split Number(x=w340) -> (hi(x)=w136:u8, lo(x)=w135:u8)
  n163 = Split Number(x=w341) -> (hi(x)=w134:u8, lo(x)=w133:u8)
  n164 = Split Number(x=w421) -> ()  [unwired: 2 out]
  n165 = Split Number(x=w420) -> (hi(x)=w293:u8, lo(x)=w292:u8)
  n166 = Split Number(x=w335) -> (hi(x)=w119:u8, lo(x)=w118:u8)
  n167 = Split Number(x=w336) -> (hi(x)=w117:u8, lo(x)=w116:u8)
  n168 = Split Number(x=w333) -> (hi(x)=w115:u8, lo(x)=w114:u8)
  n169 = Split Number(x=w334) -> (hi(x)=w113:u8, lo(x)=w112:u8)
  n170 = Split Number(x=w330) -> (hi(x)=w331:u16, lo(x)=w332:u16)
  n171 = Split Number(x=w327) -> (hi(x)=w328:u16, lo(x)=w329:u16)
  n172 = Fract/Exp String To Number(string=w378) -> (number=w379:dbl)  [unwired: 3 in, 1 out]
  n173 = Split Number(x=w46) -> (hi(x)=w24:u8, lo(x)=w23:u8)
  n174 = Split Number(x=w45) -> (hi(x)=w22:u8, lo(x)=w21:u8)
  n175 = Split Number(x=w44) -> (hi(x)=w20:u8, lo(x)=w19:u8)
  n176 = Split Number(x=w43) -> (hi(x)=w18:u8, lo(x)=w17:u8)
  n177 = Split Number(x=w42) -> (hi(x)=w16:u8, lo(x)=w15:u8)
  n178 = Split Number(x=w41) -> (hi(x)=w14:u8, lo(x)=w13:u8)
  n179 = Split Number(x=w8) -> (hi(x)=w6:u8, lo(x)=w5:u8)
  n180 = Split Number(x=w7) -> (hi(x)=w4:u8, lo(x)=w3:u8)
  n181 = Split Number(x=w83) -> (hi(x)=w365:u16, lo(x)=w364:u16)
  n182 = Split Number(x=w82) -> (hi(x)=w363:u16, lo(x)=w362:u16)
  n183 = Split Number(x=w217) -> (lo(x)=w237:u16)  [unwired: 1 out]
  n184 = Split Number(x=w216) -> (hi(x)=w219:u16, lo(x)=w218:u16)
  n185 = Split Number(x=w413) -> (hi(x)=w279:u8, lo(x)=w278:u8)
  n186 = Split Number(x=w409) -> (hi(x)=w277:u8, lo(x)=w276:u8)
  n187 = Split Number(x=w408) -> (hi(x)=w275:u8, lo(x)=w274:u8)
  n188 = Split Number(x=w407) -> (hi(x)=w273:u8, lo(x)=w272:u8)
  n189 = Split Number(x=w406) -> (hi(x)=w271:u8, lo(x)=w270:u8)
  n190 = Split Number(x=w405) -> (hi(x)=w269:u8, lo(x)=w268:u8)
  n191 = Split Number(x=w401) -> (hi(x)=w267:u8, lo(x)=w266:u8)
  n192 = Split Number(x=w402) -> (hi(x)=w2:u8, lo(x)=w1:u8)
  n193 = To Unsigned Long Integer(number=w379) -> (unsigned 32bit integer=w377:u32)
  n194 = Split Number(x=w264) -> (hi(x)=w254:u8, lo(x)=w253:u8)
  n195 = Split Number(x=w263) -> (hi(x)=w252:u8, lo(x)=w251:u8)
  n196 = Split Number(x=w262) -> (hi(x)=w250:u8, lo(x)=w249:u8)
  n197 = Split Number(x=w261) -> (hi(x)=w248:u8, lo(x)=w247:u8)
  n198 = Split Number(x=w260) -> (hi(x)=w246:u8, lo(x)=w245:u8)
  n199 = Split Number(x=w259) -> (hi(x)=w244:u8, lo(x)=w243:u8)
  n200 = Split Number(x=w258) -> (hi(x)=w242:u8, lo(x)=w241:u8)
  n201 = Split Number(x=w257) -> (hi(x)=w240:u8, lo(x)=w239:u8)
  n202 = Split Number(x=w374) -> (hi(x)=w428:u16, lo(x)=w429:u16)
  n203 = Split Number(x=w377) -> (hi(x)=w433:u16, lo(x)=w432:u16)
  n204 = To Unsigned Byte Integer(number=w223) -> (unsigned 8bit integer=w211:u8)
  n205 = Split Number(x=w331) -> (hi(x)=w111:u8, lo(x)=w110:u8)
  n206 = Split Number(x=w332) -> (hi(x)=w109:u8, lo(x)=w108:u8)
  n207 = Split Number(x=w328) -> (hi(x)=w107:u8, lo(x)=w106:u8)
  n208 = Split Number(x=w329) -> (hi(x)=w105:u8, lo(x)=w104:u8)
  n209 = To Unsigned Byte Integer(number=w224) -> (unsigned 8bit integer=w212:u8)
  n210 = Split Number(x=w237) -> (hi(x)=w202:u8, lo(x)=w201:u8)
  n211 = Split Number(x=w219) -> (hi(x)=w200:u8, lo(x)=w199:u8)
  n212 = Split Number(x=w218) -> (hi(x)=w198:u8, lo(x)=w197:u8)
  n213 = Split Number(x=w365) -> (hi(x)=w210:u8, lo(x)=w209:u8)
  n214 = Split Number(x=w364) -> (hi(x)=w208:u8, lo(x)=w207:u8)
  n215 = Split Number(x=w363) -> (hi(x)=w206:u8, lo(x)=w205:u8)
  n216 = Split Number(x=w362) -> (hi(x)=w204:u8, lo(x)=w203:u8)
  n217 = To Unsigned Byte Integer(number=w423) -> (unsigned 8bit integer=w295:u8)
  n218 = To Unsigned Byte Integer(number=w422) -> (unsigned 8bit integer=w294:u8)
  n219 = Split Number(x=w428) -> (hi(x)=w291:u8, lo(x)=w290:u8)
  n220 = Split Number(x=w429) -> (hi(x)=w289:u8, lo(x)=w288:u8)
  n221 = Split Number(x=w433) -> (hi(x)=w300:u8, lo(x)=w299:u8)
  n222 = Split Number(x=w432) -> (hi(x)=w298:u8, lo(x)=w297:u8)
  n223 = To Unsigned Byte Integer(number=w380) -> (unsigned 8bit integer=w286:u8)
  n224 = To Unsigned Byte Integer(number=w381) -> (unsigned 8bit integer=w287:u8)
  n225 = To Unsigned Byte Integer(number=w384) -> (unsigned 8bit integer=w296:u8)
  n226 = Compound Arithmetic op=ADD(w300, w299, w298, w297, w296, w295, w294, w291, w290, w289, w288, w287, w286, w293, w292) -> (w285:u8)
  n227 = Compound Arithmetic op=ADD(w279, w278, w277, w276, w275, w274, w273, w272, w271, w270, w269, w268, w267, w266, w2, w1) -> (w281:u8)
  n228 = Subtract(x=u8 255, y=w281) -> (x-y=w265:u8)
  n229 = Bundle By Name(cluster=T9 {"Packet ID"=0, "Acc X_H_Cal"=0, "Acc X_L_Cal"=0, "Acc Y_H_Cal"=0, "Acc Y_L_Cal"=0, "Acc Z_H_Cal"=0, "Acc Z_L_Cal"=0, "Gyro X_H_Cal"=0, "Gyro X_L_Cal"=0, "Gyro Y_H_Cal"=0, "Gyro Y_L_Cal"=0, "Gyro Z_H_Cal"=0, "Gyro Z_L_Cal"=0, "Voltage H 3.1V"=0, "Voltage L 3.1V"=0, "Voltage H 2.8V"=0, "Voltage L 2.8V"=0, "Check sum"=0} ("Cal information"), "Packet ID"=u8 131, "Acc X_H_Cal"=w279, "Acc X_L_Cal"=w278, "Acc Y_H_Cal"=w277, "Acc Y_L_Cal"=w276, "Acc Z_H_Cal"=w275, "Acc Z_L_Cal"=w274, "Gyro X_H_Cal"=w273, "Gyro X_L_Cal"=w272, "Gyro Y_H_Cal"=w271, "Gyro Y_L_Cal"=w270, "Gyro Z_H_Cal"=w269, "Gyro Z_L_Cal"=w268, "Voltage H 3.1V"=w267, "Voltage L 3.1V"=w266, "Voltage H 2.8V"=w2, "Voltage L 2.8V"=w1, "Check sum"=w265) -> (→"Cal information":T9)
  n230 = Compound Arithmetic op=ADD(w254, w253, w252, w251, w250, w249, w248, w247, w246, w245, w244, w243, w242, w241, w240, w239) -> (w255:u8)
  n231 = Subtract(x=u8 255, y=w255) -> (x-y=w238:u8)
  n232 = Compound Arithmetic op=ADD(w212, w211, w210, w209, w208, w207, w206, w205, w204, w203, w202, w201, w200, w199, w198, w197) -> (w214:u8)
  n233 = Compound Arithmetic op=ADD(w148, w147, w146, w145, w144, w143, w142, w141, w140, w139, w138, w137, w136, w135, w134, w133) -> (w150:u8)
  n234 = Bundle By Name(cluster=T8 {"Packet ID"=0, "Sensor 1_H"=0, "Sensor 1_L"=0, "Sensor 2_H"=0, "Sensor 2_L "=0, "Sensor 3_H"=0, "Sensor 3_L"=0, "Sensor 4_H"=0, "Sensor 4_L"=0, "Sensor 5_H"=0, "Sensor 5_L"=0, "Sensor 6_H"=0, "Sensor 6_L"=0, "Sensor 7_H"=0, "Sensor 7_L"=0, "Sensor 8_H"=0, "Sensor 8_L"=0, "Check sum"=0} ("PCAP zero information"), "Packet ID"=u8 136, "Sensor 1_H"=w254, "Sensor 1_L"=w253, "Sensor 2_H"=w252, "Sensor 2_L"=w251, "Sensor 3_H"=w250, "Sensor 3_L"=w249, "Sensor 4_H"=w248, "Sensor 4_L"=w247, "Sensor 5_H"=w246, "Sensor 5_L"=w245, "Sensor 6_H"=w244, "Sensor 6_L"=w243, "Sensor 7_H"=w242, "Sensor 7_L"=w241, "Sensor 8_H"=w240, "Sensor 8_L"=w239, "Check sum"=w238) -> (→"PCAP zero information":T8)
  n235 = Compound Arithmetic op=ADD(w300, w299, w298, w297, w296, w295, w294, w293, w292, w291, w290, w289, w288, w287, w286, w285) -> (w283:u8)
  n236 = Subtract(x=u8 255, y=w214) -> (x-y=w213:u8)
  n237 = Subtract(x=u8 255, y=w150) -> (x-y=w149:u8)
  n238 = Compound Arithmetic op=ADD(w180, w179, w178, w177, w176, w175, w174, w173, w172, w171, w170, w169, w168, w167, w166, w165) -> (w182:u8)
  n239 = Compound Arithmetic op=ADD(w119, w118, w117, w116, w115, w114, w113, w112, w111, w110, w109, w108, w107, w106, w105, w104) -> (w121:u8)
  n240 = Bundle By Name(cluster=T6 {"Packet ID"=0, "Firmware Revision"=0, "Operative Side"=0, "Cal_Compart. A_10_1"=0, "Cal_Compart. A_10_2"=0, "Cal_Compart. A_10_3"=0, "Cal_Compart. A_10_4"=0, "Cal_Compart. B_10_1"=0, "Cal_Compart. B_10_2"=0, "Cal_Compart. B_10_3"=0, "Cal_Compart. B_10_4"=0, "Reserved_1"=0, "Reserved_2"=0, "Reserved_3"=0, "Reserved_4"=0, "Reserved_5"=0, "Reserved_6"=0, "Check sum"=0} ("Cal information"), "Packet ID"=u8 145, "Firmware Revision"=w212, "Operative Side"=w211, "Cal_Compart. A_10_1"=w210, "Cal_Compart. A_10_2"=w209, "Cal_Compart. A_10_3"=w208, "Cal_Compart. A_10_4"=w207, "Cal_Compart. B_10_1"=w206, "Cal_Compart. B_10_2"=w205, "Cal_Compart. B_10_3"=w204, "Cal_Compart. B_10_4"=w203, "Reserved_1"=w202, "Reserved_2"=w201, "Reserved_3"=w200, "Reserved_4"=w199, "Reserved_5"=w198, "Reserved_6"=w197, "Check sum"=w213) -> (→"data1":T6)
  n241 = Subtract(x=u8 255, y=w283) -> (x-y=w282:u8)
  n242 = Bundle By Name(cluster=T4 {"Packet ID"=0, "Cal_Compart. A_13_1"=0, "Cal_Compart. A_13_2"=0, "Cal_Compart. A_13_3"=0, "Cal_Compart. A_13_4"=0, "Cal_Compart. B_13_1"=0, "Cal_Compart. B_13_2"=0, "Cal_Compart. B_13_3"=0, "Cal_Compart. B_13_4"=0, "Cal_Compart. A_14_1"=0, "Cal_Compart. A_14_2"=0, "Cal_Compart. A_14_3"=0, "Cal_Compart. A_14_4"=0, "Cal_Compart. B_14_1"=0, "Cal_Compart. B_14_2"=0, "Cal_Compart. B_14_3"=0, "Cal_Compart. B_14_4"=0, "Check sum"=0} ("Cal information"), "Packet ID"=u8 148, "Cal_Compart. A_13_1"=w148, "Cal_Compart. A_13_2"=w147, "Cal_Compart. A_13_3"=w146, "Cal_Compart. A_13_4"=w145, "Cal_Compart. B_13_1"=w144, "Cal_Compart. B_13_2"=w143, "Cal_Compart. B_13_3"=w142, "Cal_Compart. B_13_4"=w141, "Cal_Compart. A_14_1"=w140, "Cal_Compart. A_14_2"=w139, "Cal_Compart. A_14_3"=w138, "Cal_Compart. A_14_4"=w137, "Cal_Compart. B_14_1"=w136, "Cal_Compart. B_14_2"=w135, "Cal_Compart. B_14_3"=w134, "Cal_Compart. B_14_4"=w133, "Check sum"=w149) -> (→"data3":T4)
  n243 = Bundle By Name(cluster=T7 {"Packet ID"=0, "Device ID 1"=0, "Device ID 2"=0, "Device ID 3"=0, "Device ID 4"=0, "Year"=0, "Month"=0, "Day"=0, "Device Type H"=0, "Device Type L"=0, "Manufacturer Lot ID 1"=0, "Manufacturer Lot ID 2"=0, "Manufacturer Lot ID 3"=0, "Manufacturer Lot ID 4"=0, "Scale A"=0, "Scale B"=0, "Check sum"=0, "Check sum 2"=0} ("Device information"), "Packet ID"=u8 129, "Device ID 1"=w300, "Device ID 2"=w299, "Device ID 3"=w298, "Device ID 4"=w297, "Year"=w296, "Month"=w295, "Day"=w294, "Device Type H"=w293, "Device Type L"=w292, "Manufacturer Lot ID 1"=w291, "Manufacturer Lot ID 2"=w290, "Manufacturer Lot ID 3"=w289, "Manufacturer Lot ID 4"=w288, "Scale A"=w287, "Scale B"=w286, "Check sum"=w285, "Check sum 2"=w282) -> (→"Device information":T7)
  n244 = Compound Arithmetic op=ADD(w62, w61, w60, w59, w58, w57, w56, w55, w54, w53, w52, w51, w50, w49, w48, w47) -> (w64:u8)
  n245 = Subtract(x=u8 255, y=w182) -> (x-y=w181:u8)
  n246 = Subtract(x=u8 255, y=w121) -> (x-y=w120:u8)
  n247 = Bundle By Name(cluster=T5 {"Packet ID"=0, "Cal_Compart. A_11_1"=0, "Cal_Compart. A_11_2"=0, "Cal_Compart. A_11_3"=0, "Cal_Compart. A_11_4"=0, "Cal_Compart. B_11_1"=0, "Cal_Compart. B_11_2"=0, "Cal_Compart. B_11_3"=0, "Cal_Compart. B_11_4"=0, "Cal_Compart. A_12_1"=0, "Cal_Compart. A_12_2"=0, "Cal_Compart. A_12_3"=0, "Cal_Compart. A_12_4"=0, "Cal_Compart. B_12_1"=0, "Cal_Compart. B_12_2"=0, "Cal_Compart. B_12_3"=0, "Cal_Compart. B_12_4"=0, "Check sum"=0} ("Cal information"), "Packet ID"=u8 146, "Cal_Compart. A_11_1"=w180, "Cal_Compart. A_11_2"=w179, "Cal_Compart. A_11_3"=w178, "Cal_Compart. A_11_4"=w177, "Cal_Compart. B_11_1"=w176, "Cal_Compart. B_11_2"=w175, "Cal_Compart. B_11_3"=w174, "Cal_Compart. B_11_4"=w173, "Cal_Compart. A_12_1"=w172, "Cal_Compart. A_12_2"=w171, "Cal_Compart. A_12_3"=w170, "Cal_Compart. A_12_4"=w169, "Cal_Compart. B_12_1"=w168, "Cal_Compart. B_12_2"=w167, "Cal_Compart. B_12_3"=w166, "Cal_Compart. B_12_4"=w165, "Check sum"=w181) -> (→"data2":T5)
  n248 = Bundle By Name(cluster=T3 {"Packet ID"=0, "Cal_Compart. A_16_1"=0, "Cal_Compart. A_16_2"=0, "Cal_Compart. A_16_3"=0, "Cal_Compart. A_16_4"=0, "Cal_Compart. B_16_1"=0, "Cal_Compart. B_16_2"=0, "Cal_Compart. B_16_3"=0, "Cal_Compart. B_16_4"=0, "Reserved_1"=0, "Reserved_2"=0, "Reserved_3"=0, "Reserved_4"=0, "Reserved_5"=0, "Reserved_6"=0, "Reserved_7"=0, "Reserved_8"=0, "Check sum"=0} ("Cal information"), "Packet ID"=u8 152, "Cal_Compart. A_16_1"=w119, "Cal_Compart. A_16_2"=w118, "Cal_Compart. A_16_3"=w117, "Cal_Compart. A_16_4"=w116, "Cal_Compart. B_16_1"=w115, "Cal_Compart. B_16_2"=w114, "Cal_Compart. B_16_3"=w113, "Cal_Compart. B_16_4"=w112, "Reserved_1"=w111, "Reserved_2"=w110, "Reserved_3"=w109, "Reserved_4"=w108, "Reserved_5"=w107, "Reserved_6"=w106, "Reserved_7"=w105, "Reserved_8"=w104, "Check sum"=w120) -> (→"data4":T3)
  n249 = Subtract(x=u8 255, y=w64) -> (x-y=w63:u8)
  n250 = Compound Arithmetic op=ADD(w24, w23, w22, w21, w20, w19, w18, w17, w16, w15, w14, w13, w6, w5, w4, w3) -> (w26:u8)
  n251 = Bundle By Name(cluster=T2 {"Packet ID"=0, "Acc. X_0 val_H"=0, "Acc. X_0 val_L"=0, "Acc. Y_0 val_H"=0, "Acc. Y_0 val_L"=0, "Acc. Z_0 val_H"=0, "Acc. Z_0 val_L"=0, "Acc. X_45 val_H"=0, "Acc. X_45 val_L"=0, "Acc. Y_45 val_H"=0, "Acc. Y_45 val_L"=0, "Acc. Z_45 val_H"=0, "Acc. Z_45 val_L"=0, "Reserved_1"=0, "Reserved_2"=0, "Reserved_3"=0, "Reserved_4"=0, "Check sum"=0} ("Cal information"), "Packet ID"=u8 161, "Acc. X_0 val_H"=w62, "Acc. X_0 val_L"=w61, "Acc. Y_0 val_H"=w60, "Acc. Y_0 val_L"=w59, "Acc. Z_0 val_H"=w58, "Acc. Z_0 val_L"=w57, "Acc. X_45 val_H"=w56, "Acc. X_45 val_L"=w55, "Acc. Y_45 val_H"=w54, "Acc. Y_45 val_L"=w53, "Acc. Z_45 val_H"=w52, "Acc. Z_45 val_L"=w51, "Reserved_1"=w50, "Reserved_2"=w49, "Reserved_3"=w48, "Reserved_4"=w47, "Check sum"=w63) -> (→"Acclerometer value(0, 45)":T2)
  n252 = Subtract(x=u8 255, y=w26) -> (x-y=w25:u8)
  n253 = Bundle By Name(cluster=T1 {"Packet ID"=0, "Acc. X_90 val_H"=0, "Acc. X_90 val_L"=0, "Acc. Y_90 val_H"=0, "Acc. Y_90 val_L"=0, "Acc. Z_90 val_H"=0, "Acc. Z_90 val_L"=0, "Acc. X_180 val_H"=0, "Acc. X_180 val_L"=0, "Acc. Y_180 val_H"=0, "Acc. Y_180 val_L"=0, "Acc. Z_180 val_H"=0, "Acc. Z_180 val_L"=0, "second counter_1"=0, "second counter_2"=0, "Reserved_1"=0, "Reserved_2"=0, "Check sum"=0} ("Cal information"), "Packet ID"=u8 163, "Acc. X_90 val_H"=w24, "Acc. X_90 val_L"=w23, "Acc. Y_90 val_H"=w22, "Acc. Y_90 val_L"=w21, "Acc. Z_90 val_H"=w20, "Acc. Z_90 val_L"=w19, "Acc. X_180 val_H"=w18, "Acc. X_180 val_L"=w17, "Acc. Y_180 val_H"=w16, "Acc. Y_180 val_L"=w15, "Acc. Z_180 val_H"=w14, "Acc. Z_180 val_L"=w13, "second counter_1"=w6, "second counter_2"=w5, "Reserved_1"=w4, "Reserved_2"=w3, "Check sum"=w25) -> (→"Acclerometer value(90, 180)":T1)
  n254 = disable-structure shown="비활성화" {
    frame Disabled {
      n255 = Hexadecimal String To Number() -> (number=w442:u32)  [unwired: 3 in, 1 out]
      n256 = To Unsigned Byte Integer(number=w442) -> ()  [unwired: 1 out]
    }
    frame Enabled {
    }
  }
